vi "Change configuration state.vi"(8 "error in":errorcluster, 9 "Enter/(leave)":bool, 10 "Address":u8, 11 "Module ID":i32=-1) -> (0 "error out":errorcluster)   [LabVIEW 2020, in "FCR100.lvlib"]
doc: "Request to enter/leave configuration state.\n_____\nCreated using DQMH Event Scripter 6.1.0.128."
uses:
  FCR100.lvlib
  Change configuration state Argument--cluster.ctl
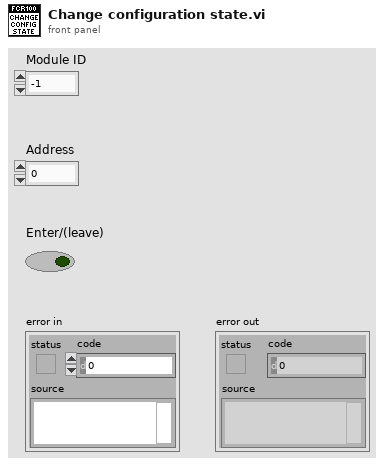
[diagram p1: front panel]
types:
  T1 = typedef "FCR100.lvlib/Change configuration state Argument--cluster.ctl" = cluster{"Module ID":i32, "Enter/(leave)":bool, "Address":u8}
  T2 = typedef "FCR100.lvlib/Request Events--cluster.ctl" = cluster{"Stop Module":refnum<user-event>, "Show Panel":refnum<user-event>, "Hide Panel":refnum<user-event>, "Show Diagram":refnum<user-event>, "Get Module Execution Status":refnum<user-event>, "Connect with dialog":refnum<user-event>, "Change configuration state":refnum<user-event>, "Change disable state":refnum<user-event>, "Search Home":refnum<user-event>, "Stop movement":refnum<user-event>, "Get state":refnum<user-event>, "Set acceleration":refnum<user-event>, "Get acceleration":refnum<user-event>, "Set velocity":refnum<user-event>, "Get velocity":refnum<user-event>, "Get ETA":refnum<user-event>, "Move absolute":refnum<user-event>, "Move relative":refnum<user-event>, "Get current position":refnum<user-event>}
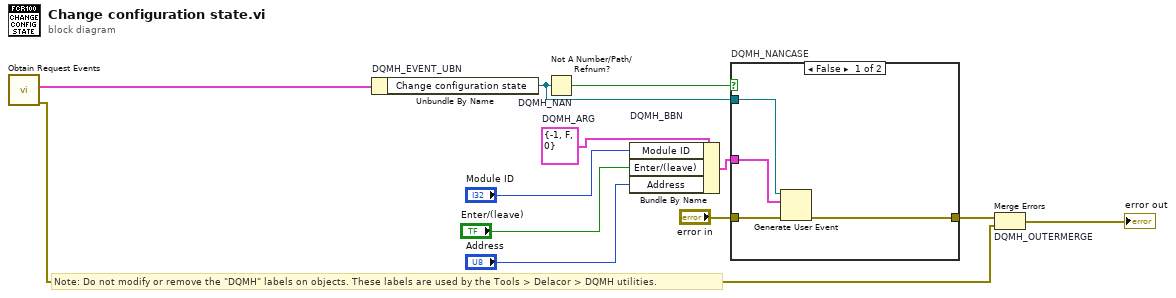
[diagram p0: block diagram]
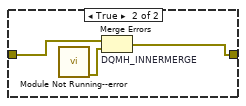
[diagram p2: hidden frame]
diagram:
  w6 = T1 {"Module ID"=-1, "Enter/(leave)"=FALSE, "Address"=0}  # DQMH_ARG
  # "Note: Do not modify or remove the \"DQMH\" labels on objects. These labels are used by the Tools > Delacor > DQMH utilities."
  n1 = call "Obtain Request Events.vi"() -> ("error out"=w3:errorcluster, "FCR100 Request Events"=w2:T2)  [unwired: 10 in]
  n2 = Unbundle By Name "DQMH_EVENT_UBN"(w2) -> ("Change configuration state"=w8:refnum<user-event>)
  n3 = Not A Number/Path/Refnum? "DQMH_NAN"(number/path/refnum=w8) -> (NaN/Path/Refnum?=w9:bool)
  n4 = Bundle By Name "DQMH_BBN"(cluster=w6, "Module ID"="Module ID", "Enter/(leave)"="Enter/(leave)", "Address"="Address") -> (w10:T1)
  n5 = case "DQMH_NANCASE" shown="False" w9 {
    tunnel: "error in" -> [w16 w19]
    tunnel: [w15 w18] -> w7
    tunnel: w8 -> [w14 _]
    tunnel: w10 -> [w13 _]
    frame False {
      n6 = Generate User Event(user event=w14, event data cluster=w13, error in=w16) -> (error out=w15:errorcluster)  [unwired: 1 in, 1 out]
    }
    frame True {
      n7 = call "Module Not Running--error.vi"() -> ("error out"=w17:errorcluster)  [unwired: 11 in]
      n8 = Merge Errors "DQMH_INNERMERGE"(w19, w17) -> (w18:errorcluster)
    }
  }
  n9 = Merge Errors "DQMH_OUTERMERGE"(w7, w3) -> (→"error out":errorcluster)
